vi "DestroySEQ.vi"(11 "FPGA out":refnum<queue>) -> ()   [LabVIEW 2019, in "FPGA.lvlib"]
uses:
  FPGA.lvlib
  FPGA.ctl
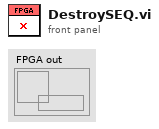
[diagram p1: front panel]
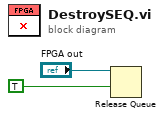
[diagram p0: block diagram]
diagram:
  n1 = Release Queue(queue="FPGA out", force destroy? (F)=TRUE) -> ()  [unwired: 1 in, 3 out]
